vi "FIR Windowed (Uniform) Filter.vi"(2 "taps":i32=25, 3 "filter type":T1(ring), 4 "high cutoff freq: fh":dbl=0.45 format="%0.2f", 5 "low cutoff freq: fl":dbl=0.125 format="%0.2f", 6 "sampling freq: fs":dbl=1.0 format="%0.2f", 7 "X":dbl[](array[numeric]) format="%0.2f") -> (0 "error":i32, 1 "Filtered Data":dbl[](array[numeric]) format="%0.2f")   [LabVIEW 2018, in "NI_AALBase.lvlib"]
doc: "Filters the input sequence using an FIR filter model."
uses:
  NI_AALBase.lvlib
  1D Convolution (DBL).vi
  NI_AALPro.lvlib
panel:
  # "FIR Windowed (Uniform) Filter"
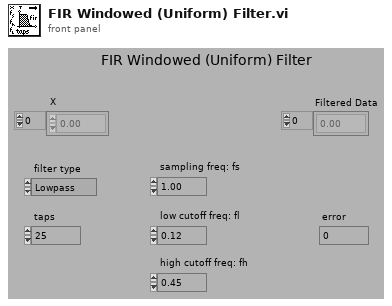
[diagram p1: front panel]
types:
  T1 = enum32{"Lowpass", "Highpass", "Bandpass", "Bandstop"}
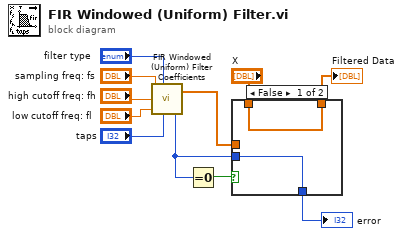
[diagram p0: block diagram]
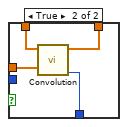
[diagram p2: hidden frame]
diagram:
  n1 = call "FIR Windowed (Uniform) Filter Coefficients.vi"("sampling freq: fs"="sampling freq: fs", "filter type"="filter type", "high cutoff freq: fh"="high cutoff freq: fh", "low cutoff freq: fl"="low cutoff freq: fl", "taps"="taps") -> ("FIR Coefficients"=w3:dbl[], "error"=w2:i32)
  n2 = Equal To 0?(x=w2) -> (x = 0?=w1:bool)
  n3 = case shown="False" w1 {
    tunnel: [w13 w15] -> w6
    tunnel: w2 -> [w13 _]
    tunnel: "X" -> [w12 w17]
    tunnel: [w12 w16] -> w4
    tunnel: w3 -> [_ w14]
    frame False {
    }
    frame True {
      n4 = call-poly "Convolution.vi"("Y"=w14, "X"=w17) -> ("error"=w15:i32, "X * Y"=w16:dbl[])  [unwired: 8 in]
    }
  }
  "Filtered Data" <- w4
  "error" <- w6
